vi "MakeToTargetCode.vi"(5 "ControlInput":string, 10 "TargetStandoff":dbl=5.0, 11 "TTarget":dbl=20.0 min=0.0 max=30.0) -> (3 "ToAmbient":string="define onecycle (pwm=100 run pwmloop 5A.PID.Setpoint=-131.500000  while(#3C >-129.5){pause 0.2 s}pwm=10 pause 10 min kill pwmloop pwm=0 relays=0 5A.PID.SetPoint=51.0 while(#3C<50.0){pause 0.2 s} pause 10 min)")   [LabVIEW 2024]
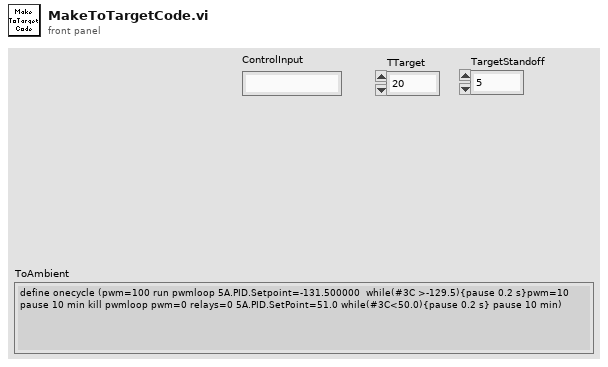
[diagram p1: front panel]
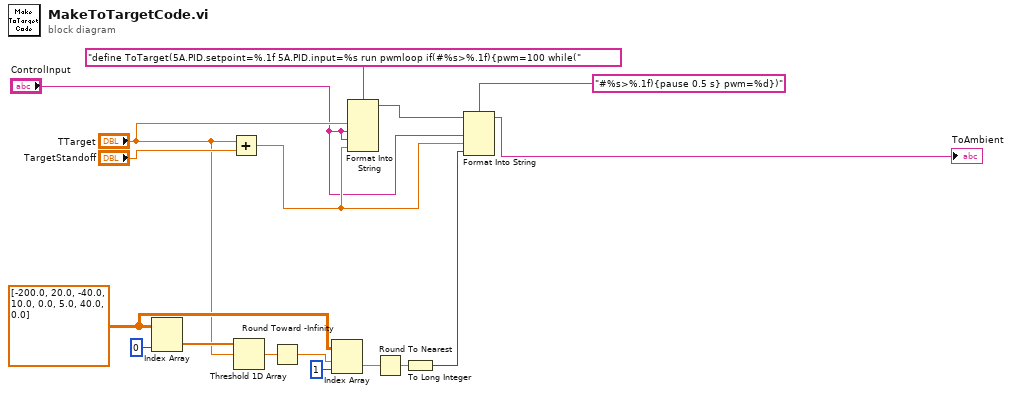
[diagram p0: block diagram]
diagram:
  w9 = dbl[][] [[-200.0, 20.0], [-40.0, 10.0], [0.0, 5.0], [40.0, 0.0]]
  n1 = Index Array(array=w9, index (col)=0 ("disabled index (col)")) -> (element=w10:dbl[])  [unwired: 1 in]
  n2 = Add(x="TTarget", y="TargetStandoff") -> (x+y=w12:dbl)
  n3 = Threshold 1D Array(2:"TTarget", 3:w10) -> (0:w7:dbl)  [unwired: 1 in]
  n4 = Round Toward -Infinity(1:w7) -> (0:w6:dbl)
  n5 = Index Array(array=w9, index (row)=w6, index (col)=1 ("disabled index (col)")) -> (element=w4:dbl)
  n6 = Format Into String(format string="define ToTarget(5A.PID.setpoint=%.1f 5A.PID.input=%s run pwmloop if(#%s>%.1f){pwm=100 while(", "TTarget", "ControlInput", "ControlInput", w12) -> (resulting string=w16:string)  [unwired: 2 in, 1 out]
  n7 = Round To Nearest(number=w4) -> (nearest integer value=w3:dbl)
  n8 = To Long Integer(number=w3) -> (32bit integer=w2:i32)
  n9 = Format Into String(format string="#%s>%.1f){pause 0.5 s} pwm=%d})", initial string=w16, "ControlInput", w12, w2) -> (resulting string=→"ToAmbient":string)  [unwired: 1 in, 1 out]
